vi "Set Termination.vi"(6 "Channel":i32=1, 8 "error in (no error)":errorcluster, 10 "Termination":enum16{"50_Ohm", "High_Z"}(ring), 11 "336XX in":refnum<class "336XX.lvclass">) -> (0 "error out":errorcluster, 3 "336XX out":refnum<class "336XX.lvclass">)   [LabVIEW 2019, in "336XX.lvlib" / "336XX.lvclass"]
uses:
  Library/336XX.lvclass
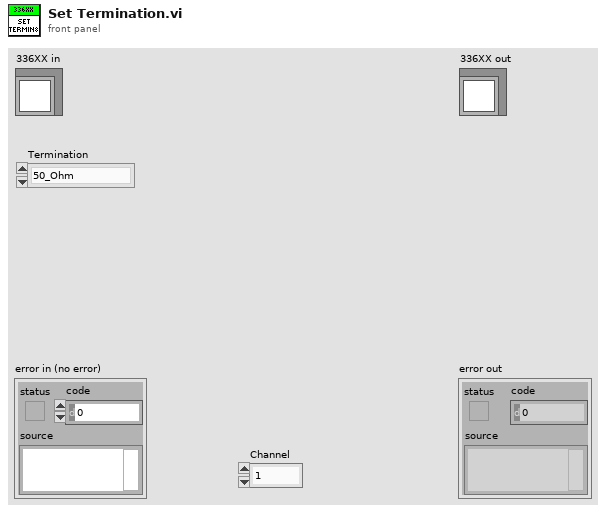
[diagram p1: front panel]
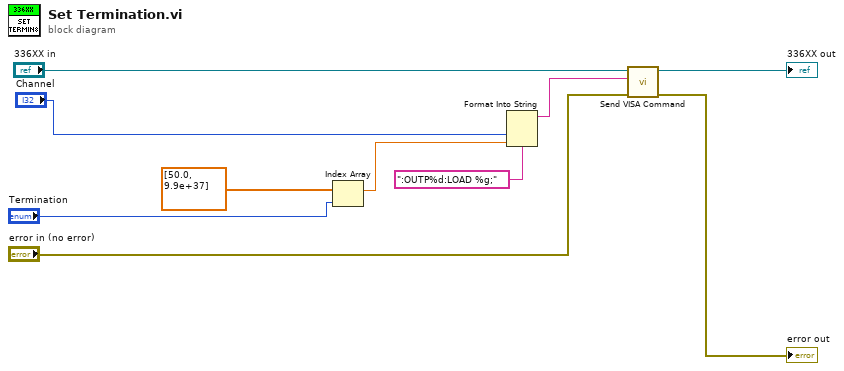
[diagram p0: block diagram]
diagram:
  n1 = Index Array(array=dbl[] [50.0, 9.9e+37], index="Termination") -> (element=w4:dbl)
  n2 = Format Into String(format string=":OUTP%d:LOAD %g;", "Channel", w4) -> (resulting string=w6:string)  [unwired: 2 in, 1 out]
  n3 = call "Send VISA Command.vi"("error in (no error)"="error in (no error)", "Command"=w6, "336XX in"="336XX in") -> ("error out"=→"error out":errorcluster, "336XX out"=→"336XX out":refnum<class "336XX.lvclass">)  [unwired: 7 in]
